vi "NISE.remote.Open Generic Command.vi"(0 "SLSC Remote in":refnum<class "SLSC Interface.lvclass">, 5 "resource":string, 7 "command in":refnum<k21>, 11 "error in (no error)":errorcluster) -> (4 "SLSC Remote out":refnum<class "SLSC Interface.lvclass">, 8 "command out":refnum<k21>, 15 "error out":errorcluster)   [LabVIEW 2016, in "SLSC Interface.lvclass"]
uses:
  SLSC Interface Class/SLSC Interface.lvclass
  SLSC Interface Class/SLSC Interface.lvclass/SLSC Interface.ctl
  SLSC Interface Class/NISE.Read client handle.vi
  SLSC Interface Class/NISE.Read URL.vi
  SLSC Interface Class/NISE.Read session.vi
  <vilib>/NI/NI JSONRPC Server Framework/Classes/Server/server.Format Client Request (Auto-Increment).vi
  <vilib>/httpClient/POSTBuffer.vi
  <vilib>/httpClient/LabVIEWHTTPClient.lvlib
  <vilib>/NI/NI JSONRPC Server Framework/Classes/Server/JSONRPC Server.lvclass
  <vilib>/NI/JSON Support for LabVIEW/JSON Value/JSON Value.lvclass
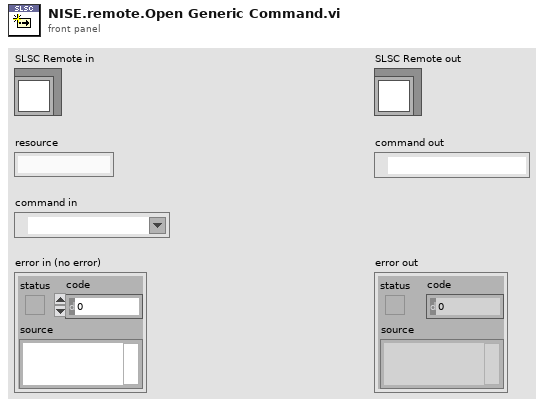
[diagram p1: front panel]
types:
  T1 = typedef "LabVIEWHTTPClient.lvlib/ClientHandle.ctl" = refnum<k1>
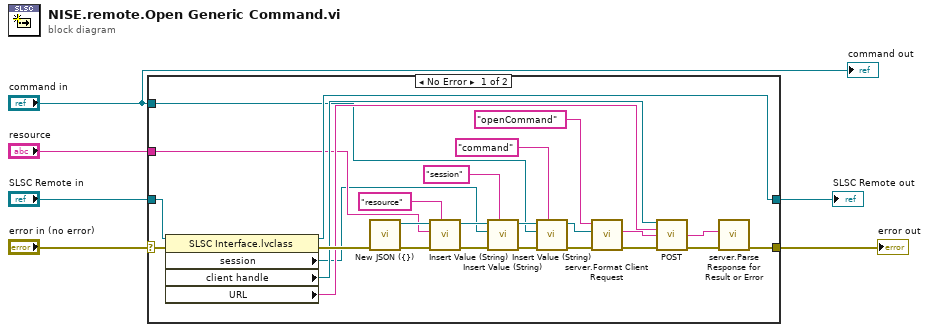
[diagram p0: block diagram]
diagram:
  n1 = case shown="No Error" "error in (no error)" {
    selector: "error in (no error)" -> [w30 w33]
    tunnel: "command in" -> [w7 _]
    tunnel: "SLSC Remote in" -> [w32 w34]
    tunnel: [w31 w34] -> w3
    tunnel: [w20 w33] -> w1
    tunnel: "resource" -> [w9 _]
    frame No Error {
      n2 = property class="SLSC Interface.lvclass"(reference=w32, error in=w30) -> (reference out=w31:refnum<class "SLSC Interface.lvclass">, error out=w29:errorcluster, "session"=w8:refnum<k21>, "client handle"=w25:T1, "URL"=w24:string)
      n3 = call <vilib>:"New JSON ({}).vi"("error in (no error)"=w29) -> ("error out"=w28:errorcluster, "JSON Value out"=w12:refnum<class "JSON Value.lvclass">)  [unwired: 9 in]
      n4 = call <vilib>:"Insert Value (String).vi"("key"="resource" ("Name"), "error in (no error)"=w28, "value"=w9, "JSON Value in"=w12) -> ("error out"=w27:errorcluster, "JSON Value out"=w11:refnum<class "JSON Value.lvclass">)  [unwired: 5 in, 1 out]
      n5 = call <vilib>:"Insert Value (String).vi"("key"="session" ("Name"), "error in (no error)"=w27, "value"=w8, "JSON Value in"=w11) -> ("error out"=w19:errorcluster, "JSON Value out"=w10:refnum<class "JSON Value.lvclass">)  [unwired: 5 in, 1 out]
      n6 = call <vilib>:"Insert Value (String).vi"("key"="command" ("Name"), "error in (no error)"=w19, "value"=w7, "JSON Value in"=w10) -> ("error out"=w17:errorcluster, "JSON Value out"=w18:refnum<class "JSON Value.lvclass">)  [unwired: 5 in, 1 out]
      n7 = call-poly <vilib>:"server.Format Client Request.vi"("error in (no error)"=w17, "JSON Value in"=w18, "method"="openCommand") -> ("error out"=w23:errorcluster, "Request String"=w26:string)  [unwired: 7 in]
      n8 = call-poly <vilib>:"POST.vi"("client handle"=w25, "url"=w24, "buffer"=w26, "error in (no error)"=w23) -> ("body"=w22:string, "error out"=w21:errorcluster)  [unwired: 8 in, 2 out]
      n9 = call <vilib>:"server.Parse Response for Result or Error.vi"("error in"=w21, "Response String In"=w22) -> ("error out"=w20:errorcluster)  [unwired: 7 in, 2 out]
    }
    frame Error {
    }
  }
  "error out" <- w1
  "SLSC Remote out" <- w3
  "command out" <- "command in"
